vi "Read Static.vi"(8 "error in (no error)":errorcluster, 11 "Level in":refnum<class "Level.lvclass">) -> (0 "error out":errorcluster, 2 "Static":cluster{"Voltage":dbl[], "Power":dbl[]}, 3 "Level out":refnum<class "Level.lvclass">)   [LabVIEW 2020, in "Level.lvclass"]
uses:
  Level.lvclass
  Level.lvclass/Level.ctl
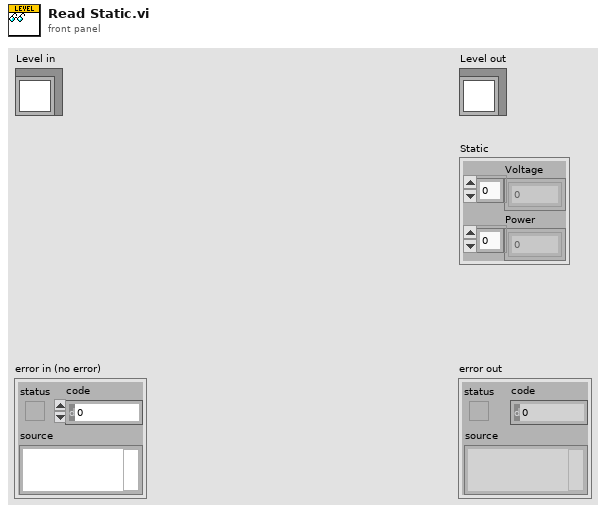
[diagram p1: front panel]
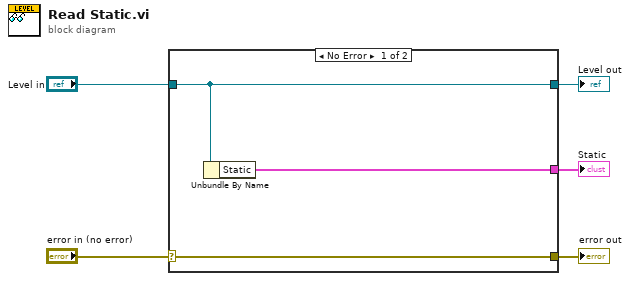
[diagram p0: block diagram]
diagram:
  n1 = case shown="No Error" "error in (no error)" {
    selector: "error in (no error)" -> [w8 w9]
    tunnel: [w8 w9] -> w4
    tunnel: [w7 w10] -> w2
    tunnel: "Level in" -> [w7 w10]
    tunnel: [w6 _] -> w1
    frame No Error {
      n2 = Unbundle By Name(w7) -> ("Static"=w6:cluster{"Voltage":dbl[], "Power":dbl[]})
    }
    frame Error {
    }
  }
  "error out" <- w4
  "Level out" <- w2
  "Static" <- w1
